vi "Start and Forget FP.vi"(8 "error in":errorcluster, 11 "GUI in":refnum<class "GUI.lvclass">) -> (0 "error out":errorcluster, 1 "Stop":refnum<user-event>, 2 "UI Ref":refnum<vi>, 3 "GUI out":refnum<class "GUI.lvclass">)   [LabVIEW 2013, in "GUI.lvclass"]
doc: "Takes the child class for GUI and starts the VI for that specific implementation called Front Panel.vi. The x8 bit for the Open VI function prepares the VI for reentrant execution."
uses:
  GUI.lvclass
  GUI.lvclass/GUI.ctl
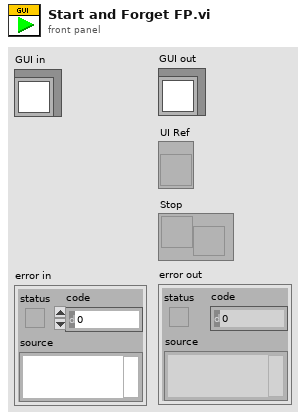
[diagram p1: front panel]
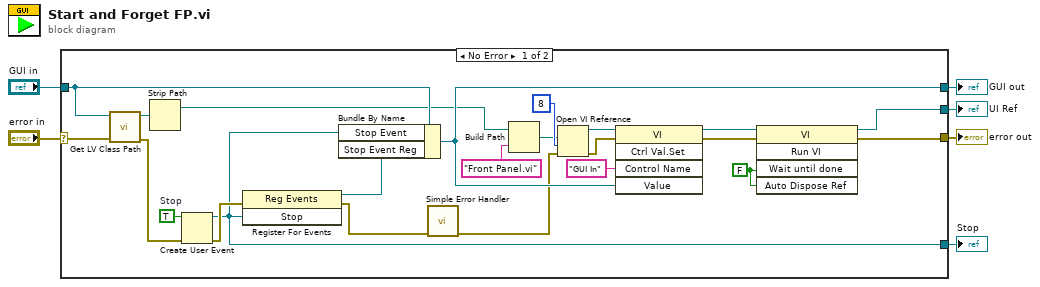
[diagram p0: block diagram]
diagram:
  n1 = case shown="No Error" "error in" {
    selector: "error in" -> [w24 w31]
    tunnel: [w21 w31] -> w5
    tunnel: [w13 w30] -> w3
    tunnel: "GUI in" -> [w16 w30]
    tunnel: [w20 _] -> w2
    tunnel: [w14 _] -> w1
    frame No Error {
      w19 = TRUE  # Stop
      w25 = FALSE ("Wait Until Done")
      n2 = call <vilib>:"Get LV Class Path.vi"("error in (no error)"=w24, "object"=w16) -> ("error out"=w18:errorcluster, "class path"=w29:path)  [unwired: 8 in]
      n3 = Strip Path(path=w29) -> (stripped path=w9:path)  [unwired: 1 out]
      n4 = Create User Event(user event datatype=w19, error in=w18) -> (user event=w14:refnum<user-event>, error out=w17:errorcluster)
      n5 = register-events(error in=w17, w14) -> (reference out=w15:refnum<event-registration>, error out=w11:errorcluster)  [unwired: 1 in]
      n6 = Bundle By Name(cluster=w16, "Stop Event"=w14, "Stop Event Reg"=w15) -> (w13:refnum<class "GUI.lvclass">)
      n7 = call <vilib>:"Simple Error Handler.vi"("error in (no error)"=w11) -> ("error out"=w10:errorcluster)  [unwired: 4 in, 4 out]
      n8 = Build Path(base path=w9, name or relative path="Front Panel.vi") -> (appended path=w7:path)
      n9 = Open VI Reference(vi path=w7, options=8, error in (no error)=w10) -> (vi reference=w27:refnum<vi>, error out=w8:errorcluster)  [unwired: 3 in]
      n10 = invoke class="VI" method="Ctrl Val.Set"(reference=w27, error in=w8, "Control Name"="GUI In", "Value"=w13) -> (reference out=w23:refnum<vi>, error out=w22:errorcluster)  [unwired: 1 in, 3 out]
      n11 = invoke class="VI" method="Run VI"(reference=w23, error in=w22, "Wait until done"=w25, "Auto Dispose Ref"=w25) -> (reference out=w20:refnum<vi>, error out=w21:errorcluster)  [unwired: 1 in, 3 out]
    }
    frame Error {
    }
  }
  "error out" <- w5
  "GUI out" <- w3
  "UI Ref" <- w2
  "Stop" <- w1
